vi "ActionVIOnDownload.vi"(5 "System Definition Dir":path, 6 "IP address":string, 7 "Details Ref":refnum<vi>, 8 "error in (no error)":errorcluster, 10 "WebDAV session in":T1, 11 "Device Item Ref in":T2 format="%.0x") -> (0 "error out":errorcluster, 2 "WebDAV session out":T1, 3 "Device Item Ref out":T2 format="%.0x")   [LabVIEW 2019, in "NI Synchronization System Explorer.lvlib"]
uses:
  NI Synchronization System Explorer.lvlib
  <vilib>/NI VeriStand/Custom Device API/Custom Device Item Ref.ctl
  <vilib>/WebDAVClient/Advanced/SessionHandle.ctl
  Engine/RT Data Cluster.ctl
  Engine/mdevClkDisc.llb/_clkDisc_session.ctl
  Shared/Compiled Data.ctl
  Shared/Connection Settings.ctl
  Shared/Mode.ctl
  Shared/External Pin.ctl
  Shared/Routes.ctl
  Shared/Route.ctl
  Shared/Time Ref Settings.ctl
  Shared/Time Reference.ctl
  Shared/IRIG Type.ctl
  Engine/timekeeper type.ctl
  Shared/Constants.vi
  <vilib>/NI VeriStand/Custom Device API/Get Item Property (String).vi
  <vilib>/NI VeriStand/Custom Device API/Custom Device API.lvlib
  Shared/NI Synchronization Shared.lvlib
  Engine/NI Synchronization Engine.lvlib
  <vilib>/Utility/SystemLogging/NI_SystemLogging.lvlib
  <vilib>/NI VeriStand/Custom Device API/Get Item Property (Boolean).vi
  <vilib>/WebDAVClient/NI_WebDAV.lvlib
panel:
  in  "missing ni-sync-remote-config message":string="The NI Synchronization custom device failed to configure clock disciplining prior to deploying the system definition. Clock disciplining may still succeed during system initialization. If the system fails to deploy, install the \"NI-Sync Remote Configuration\" software to your real-time target."
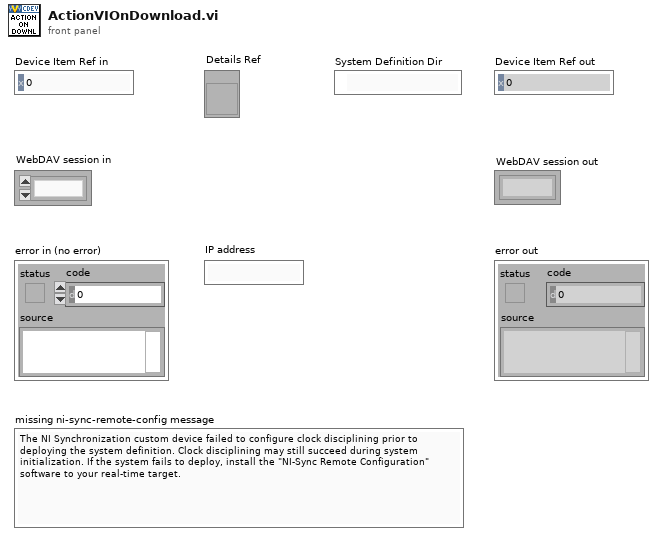
[diagram p1: front panel]
types:
  T1 = typedef "NI_WebDAV.lvlib/SessionHandle.ctl" = refnum<k1>
  T2 = typedef "Custom Device API.lvlib/Custom Device Item Ref.ctl" = u64
  T3 = typedef "NI Synchronization Engine.lvlib/RT Data Cluster.ctl" = cluster{"Timekeeper hdl":refnum<k15>, "clkDisc session":T4, "Compiled Data":T5, "OutputsData":dbl[], "OutputsFIFO":refnum<k33>, "Scan Period":u32, "Timekeeper type":T14, "SyncMod type":T14, "SyncMod hdl":refnum<k15>, "Custom Device Name":string}
  T4 = typedef "_clkDisc_session.ctl" = variant
  T5 = typedef "NI Synchronization Shared.lvlib/Compiled Data.ctl" = cluster{"SyncMod?":bool, "SyncMod":string, "ConnectionSettings":T6, "TimeKeeper":string, "ScanOffset(%)":dbl, "StartDelay(s)":u16, "Time Ref Settings":T11, "FIFO Locations":cluster{"BoardTime":i32[], "Status":i32[]}}
  T6 = typedef "NI Synchronization Shared.lvlib/Connection Settings.ctl" = cluster{"Mode":T7, "pxitrig":bool, "pfi0":bool, "pfi1":bool, "pfi2":bool, "External Pin":T8, "Routes":T9}
  T7 = typedef "NI Synchronization Shared.lvlib/Mode.ctl" = enum16{"Generate sample clock", "Route sample clock out of chassis", "Route sample clock into chassis", "Custom routes"}
  T8 = typedef "NI Synchronization Shared.lvlib/External Pin.ctl" = enum16{"PFI0", "PFI1", "PFI2"}
  T9 = typedef "NI Synchronization Shared.lvlib/Routes.ctl" = T10[]
  T10 = typedef "NI Synchronization Shared.lvlib/Route.ctl" = cluster{"Source":string, "Destination":string}
  T11 = typedef "NI Synchronization Shared.lvlib/Time Ref Settings.ctl" = cluster{"Time Reference":T12, "Priority 1":i32, "Priority 2":i32, "IRIG type":T13, "Terminal":string, "PPSSetTime":bool, "Start Time":timestamp}
  T12 = typedef "NI Synchronization Shared.lvlib/Time Reference.ctl" = enum16{"GPS", "IRIG", "PPS", "1588 Ordinary Clock", "802.1AS", "PXI Chassis Clock", "Free Running (Internal)"}
  T13 = typedef "NI Synchronization Shared.lvlib/IRIG Type.ctl" = enum16{"IRIGB DC", "IRIGB AM"}
  T14 = typedef "NI Synchronization Engine.lvlib/timekeeper type.ctl" = enum16{"6683", "6683H", "6682", "6682H", "non-timekeeper", "timekeeper"}
  T15 = typedef "Custom Device API.lvlib/Custom Device Item Info.ctl" = cluster{"Name":string, "Is Channel":bool, "GUID":string, "Is Waveform":bool}
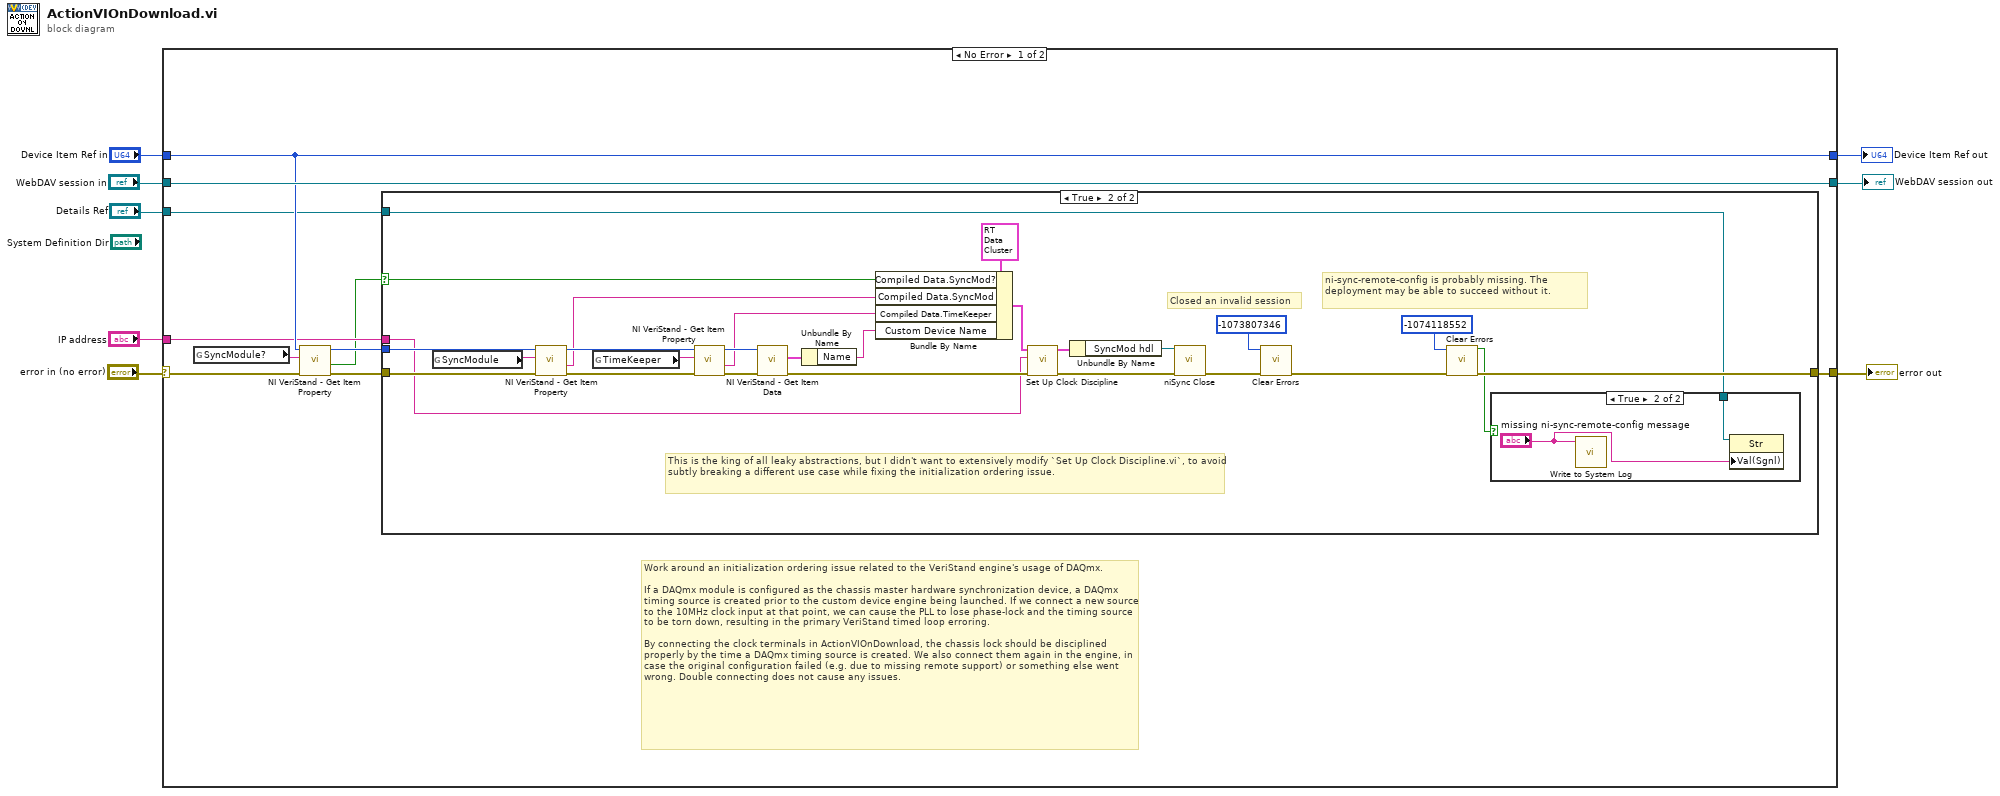
[diagram p0: block diagram]
diagram:
  n1 = case shown="No Error" "error in (no error)" {
    selector: "error in (no error)" -> [w13 w51]
    tunnel: [w11 w51] -> w7
    tunnel: "WebDAV session in" -> [w18 w50]
    tunnel: [w18 w50] -> w3
    tunnel: "Device Item Ref in" -> [w14 w49]
    tunnel: [w14 w49] -> w5
    tunnel: "IP address" -> [w12 _]
    tunnel: "Details Ref" -> [w9 _]
    frame No Error {
      # "Work around an initialization ordering issue related to the VeriStand engine's usage of DAQmx.\n\nIf a DAQmx module is configured as the chassis master hardware synchronization device, a DAQmx timing source is created prior to the custom device engine being launched. If we connect a new source to the 10MHz clock input at that point, we can cause the PLL to lose phase-lock and the timing source to be torn down, resulting in the primary VeriStand timed loop erroring.\n\nBy connecting the clock terminals in ActionVIOnDownload, the chassis lock should be disciplined properly by the time a DAQmx timing source is created. We also connect them again in the engine, in case the original configuration failed (e.g. due to missing remote support) or something else went wrong. Double connecting does not cause any issues."
      n2 = global read "Constants.vi" "SyncModule?"() -> (w15:string)
      n3 = call-poly <vilib>:"NI VeriStand - Get Item Property.vi"("error in (no error)"=w13, "Property Name"=w15, "Item Ref in"=w14) -> ("error out"=w16:errorcluster, "Value"=w10:bool, "Item Ref out"=w17:T2)  [unwired: 5 in, 1 out]
      n4 = case shown="True" w10 {
        selector: w10 -> [_ w40]
        tunnel: w17 -> [_ w46]
        tunnel: w16 -> [w19 w45]
        tunnel: w12 -> [_ w25]
        tunnel: [w19 w22] -> w11
        tunnel: w9 -> [_ w20]
        frame False {
        }
        frame True {
          # "ni-sync-remote-config is probably missing. The deployment may be able to succeed without it."
          # "This is the king of all leaky abstractions, but I didn't want to extensively modify `Set Up Clock Discipline.vi`, to avoid subtly breaking a different use case while fixing the initialization ordering issue."
          # "Closed an invalid session"
          n5 = global read "Constants.vi" "SyncModule"() -> (w44:string)
          n6 = call-poly <vilib>:"NI VeriStand - Get Item Property.vi"("error in (no error)"=w45, "Property Name"=w44, "Item Ref in"=w46) -> ("error out"=w38:errorcluster, "Value"=w26:string, "Item Ref out"=w37:T2)  [unwired: 5 in, 1 out]
          n7 = global read "Constants.vi" "TimeKeeper"() -> (w39:string)
          n8 = call-poly <vilib>:"NI VeriStand - Get Item Property.vi"("error in (no error)"=w38, "Property Name"=w39, "Item Ref in"=w37) -> ("error out"=w35:errorcluster, "Value"=w27:string, "Item Ref out"=w36:T2)  [unwired: 5 in, 1 out]
          n9 = call <vilib>:"NI VeriStand - Get Item Data.vi"("error in (no error)"=w35, "Item Ref in"=w36) -> ("error out"=w32:errorcluster, "Item Info"=w34:T15)  [unwired: 6 in, 2 out]
          n10 = Unbundle By Name(w34) -> ("Name"=w33:string)
          n11 = Bundle By Name(cluster=T3 {"Timekeeper hdl"="", "clkDisc session"=variant, "Compiled Data"={"SyncMod?"=FALSE, "SyncMod"="", "ConnectionSettings"={"Mode"=enum."Generate sample clock", "pxitrig"=FALSE, "pfi0"=FALSE, "pfi1"=FALSE, "pfi2"=FALSE, "External Pin"=enum."PFI0", "Routes"=[]}, "TimeKeeper"="", "ScanOffset(%)"=0.0, "StartDelay(s)"=0, "Time Ref Settings"={"Time Reference"=enum."GPS", "Priority 1"=0, "Priority 2"=0, "IRIG type"=enum."IRIGB AM", "Terminal"="", "PPSSetTime"=FALSE, "Start Time"=timestamp(0 s since 1904-01-01)}, "FIFO Locations"={"BoardTime"=[], "Status"=[]}}, "OutputsData"=[], "OutputsFIFO"=refnum, "Scan Period"=0, "Timekeeper type"=enum."6683", "SyncMod type"=enum."6683", "SyncMod hdl"="", "Custom Device Name"=""} ("RT Data Cluster in"), "Compiled Data.SyncMod?"=w40, "Compiled Data.SyncMod"=w26, "Compiled Data.TimeKeeper"=w27, "Custom Device Name"=w33) -> (w31:T3)
          n12 = call "Set Up Clock Discipline.vi"("error in (no error)"=w32, "Target IP Address (empty: local)"=w25, "RT Data Cluster in"=w31) -> ("error out"=w42:errorcluster, "RT Data Cluster out"=w30:T3)  [unwired: 7 in]
          n13 = Unbundle By Name(w30) -> ("SyncMod hdl"=w29:refnum<k15>)
          n14 = call <instrlib>:"niSync Close.vi"("error in (no error)"=w42, "instrument handle"=w29) -> ("error out"=w43:errorcluster)  [unwired: 9 in]
          n15 = call <vilib>:"Clear Errors.vi"("error in (no error)"=w43, "specific error code to clear (0: all)"=-1073807346) -> ("error out"=w23:errorcluster)  [unwired: 4 in, 1 out]
          n16 = call <vilib>:"Clear Errors.vi"("error in (no error)"=w23, "specific error code to clear (0: all)"=-1074118552) -> ("error out"=w22:errorcluster, "specific error cleared?"=w21:bool)  [unwired: 4 in]
          n17 = case shown="True" w21 {
            tunnel: w20 -> [_ w48]
            frame False {
            }
            frame True {
              n18 = call <vilib>:"Write to System Log.vi"("message"="missing ni-sync-remote-config message") -> ()  [unwired: 10 in, 1 out]
              n19 = property class="Str"(reference=w48, "Val(Sgnl)"="missing ni-sync-remote-config message") -> ()  [unwired: 1 in, 2 out]
            }
          }
        }
      }
    }
    frame Error {
    }
  }
  "error out" <- w7
  "Device Item Ref out" <- w5
  "WebDAV session out" <- w3
